vi "PT1000TempSensor.vi"() -> ()   [LabVIEW 2015]
uses:
  <vilib>/DAQmx/read.llb/DAQmx Read.vi
  <vilib>/DAQmx/read.llb/DAQmx Read (Analog Wfm 1Chan NSamp).vi
  <vilib>/DAQmx/miscellaneous.llb/DAQmx Fill In Error Info.vi
panel:
  out "Waveform Chart":waveform(dbl)(graph)
  out "Temp(C)":dbl(slide) scale=-10.0..100.0
  out "Temperature (Celcius)":dbl format="%#_13g"
  out "Voltage Reading":dbl format="%#_13g"
  in  "stop":bool
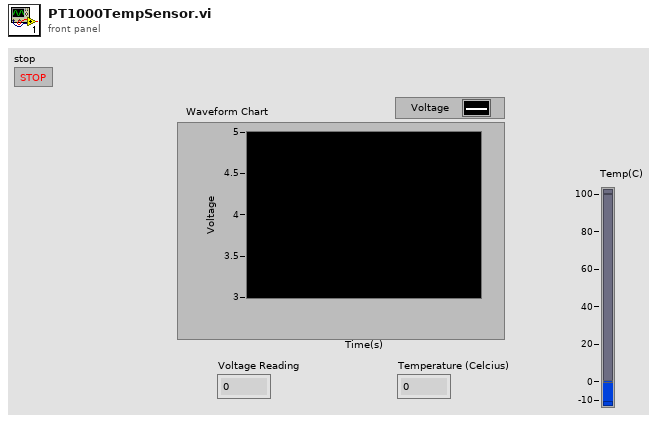
[diagram p1: front panel]
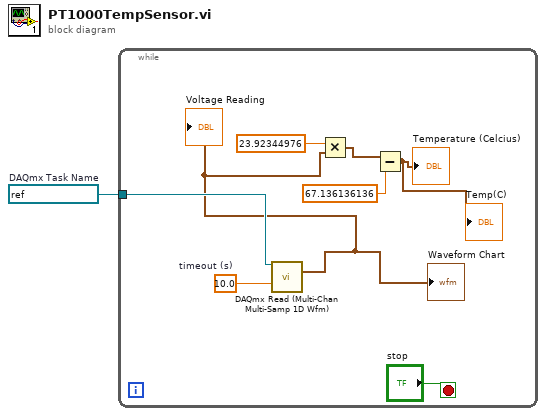
[diagram p0: block diagram]
diagram:
  w1 = refnum<k21> "AnalogInA0"  # DAQmx Task Name
  n1 = while {
    tunnel: w1 -> [w8]
    stop <- "stop" stop-if-true
    w9 = 10.0  # timeout (s)
    n2 = call-poly "DAQmx Read (Multi-Chan Multi-Samp 1D Wfm).vi"("task/channels in"=w8, "timeout"=w9) -> ("data"=w2:waveform(dbl))  [unwired: 11 in, 2 out]
    "Voltage Reading" <- w2
    "Waveform Chart" <- w2
    n3 = Multiply(x=23.92344976, y=w2) -> (x*y=w5:waveform(dbl))
    n4 = Subtract(x=w5, y=67.136136136) -> (x-y=→"Temperature (Celcius)" →"Temp(C)":waveform(dbl))
  }
